vi "ClawGetOpenClose.vi"() -> (3 "Open?":bool)   [LabVIEW 2023]
uses:
  ClawGlobal.vi
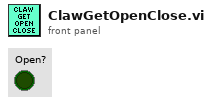
[diagram p1: front panel]
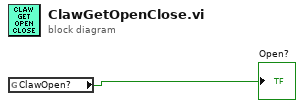
[diagram p0: block diagram]
diagram:
  n1 = global read "ClawGlobal.vi" "ClawOpen?"() -> (→"Open?":bool)
